vi "Mag Array.vi"() -> ()   [LabVIEW 2009, in "Magnet.lvclass"]
uses:
  Magnet.lvclass
panel:
  out "magarray":T1(array[cluster])
  # "this string of numbers is what I call the \"use string\" - it is a series of 4 numbers, corresponding to each scan type (wait, width, wave and magnet, in that order).  The number is converted to a binary array, which tells the computer which types of experiments within each scan type needs to be used"
  # "scan; ret"
  # "PGarm: 1 = ext, 0 = imm (cont)\nPGpatton? 1 = T, 0 = F"
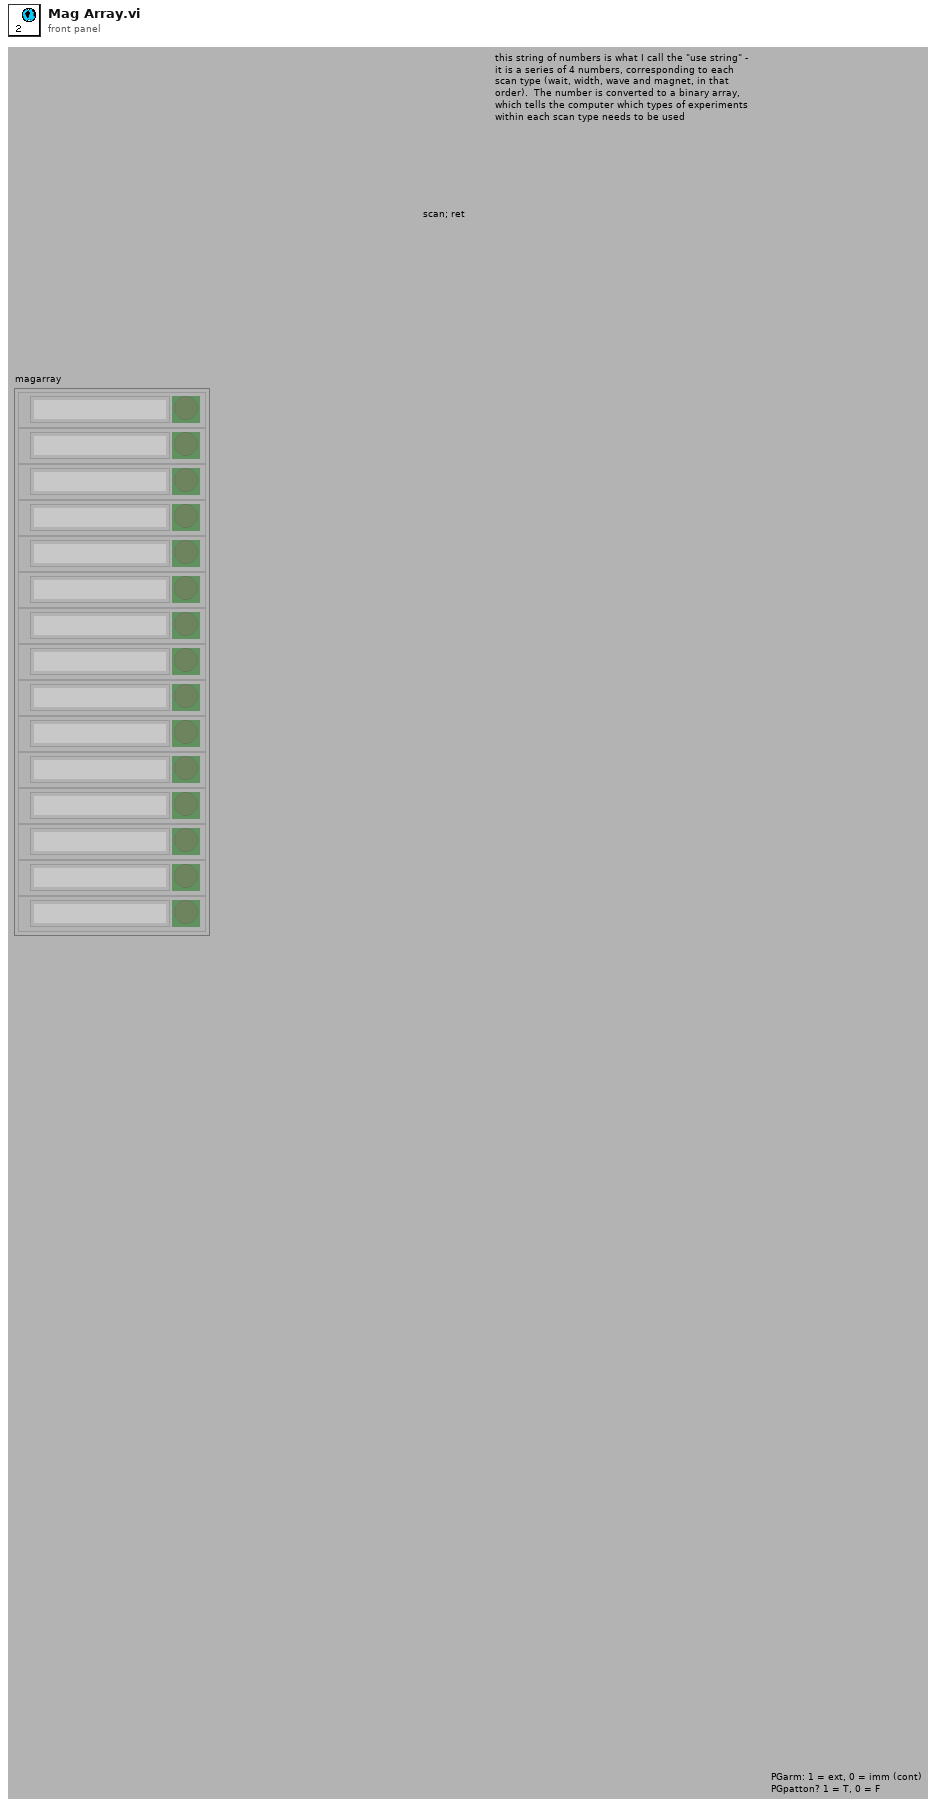
[diagram p1: front panel]
types:
  T1 = cluster{"name":string, "status":bool, "abbrev":string}[]
diagram:
